vi "Write Wvfrm Graph Reference.vi"(8 "error in (no error)":errorcluster, 10 "General Measurement UI":refnum<vi>, 11 "Measurement in":refnum<class "Measurement.lvclass">) -> (0 "error out":errorcluster, 3 "Measurement out":refnum<class "Measurement.lvclass">)   [LabVIEW 2015, in "Measurement Actor.lvlib" / "Measurement.lvclass"]
uses:
  Measurement.lvclass
  Measurement.lvclass/Measurement.ctl
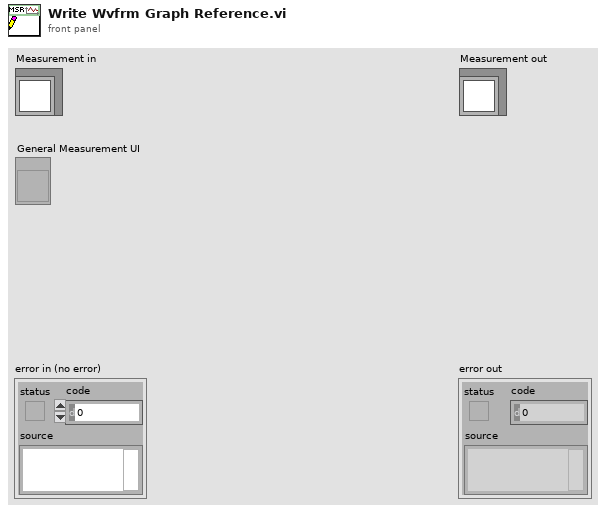
[diagram p1: front panel]
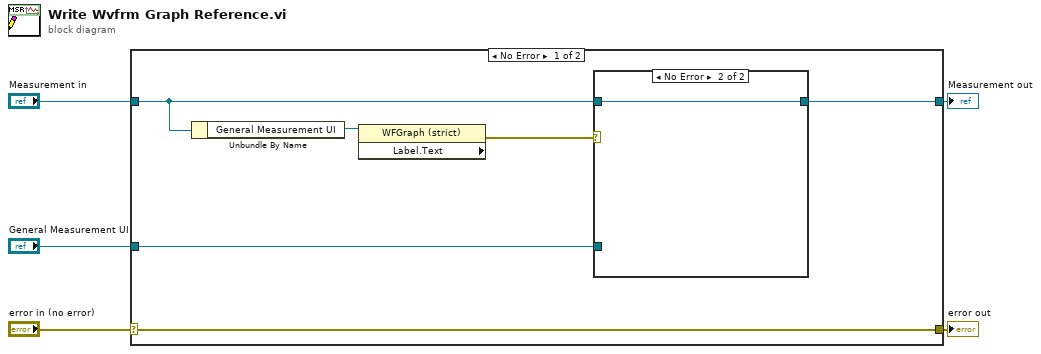
[diagram p0: block diagram]
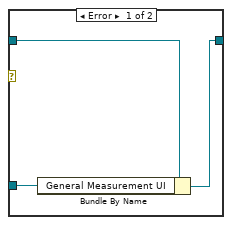
[diagram p2: hidden frame]
diagram:
  n1 = case shown="No Error" "error in (no error)" {
    selector: "error in (no error)" -> [w11 w16]
    tunnel: [w11 w16] -> w4
    tunnel: [w10 w17] -> w2
    tunnel: "Measurement in" -> [w8 w17]
    tunnel: "General Measurement UI" -> [w9 _]
    frame No Error {
      n2 = Unbundle By Name(w8) -> ("General Measurement UI"=w7:refnum<vi>)
      n3 = property class="WFGraph (strict)" props=["Label", "Text"](reference=w7) -> (error out=w6:errorcluster)  [unwired: 1 in, 2 out]
      n4 = case shown="No Error" w6 {
        tunnel: [w14 w15] -> w10
        tunnel: w9 -> [w13 _]
        tunnel: w8 -> [w12 w15]
        frame Error {
          n5 = Bundle By Name(cluster=w12, "General Measurement UI"=w13) -> (w14:refnum<class "Measurement.lvclass">)
        }
        frame No Error {
        }
      }
    }
    frame Error {
    }
  }
  "error out" <- w4
  "Measurement out" <- w2
